vi "calculate bearing example.vi"() -> ()   [LabVIEW 2011]
uses:
  <vilib>/robotics/Controls/Compass Indicator/Compass Indicator.xctl
  <vilib>/express/express arith-compare/Formula/XNode/ExpressFormulaBlockNode.xnode
panel:
  out "Result 2":dbl
  out "Result":dbl
  in  "stop":bool
  in  "Dlong2":dbl format="%#_16g"
  in  "Dlat2":dbl format="%#_16g"
  in  "Dlong1":dbl format="%#_16g"
  in  "Dlat1":dbl format="%#_16g"
  out "Final Bearing":dbl(xcontrol)
  out "Initial Bearing":dbl(xcontrol)
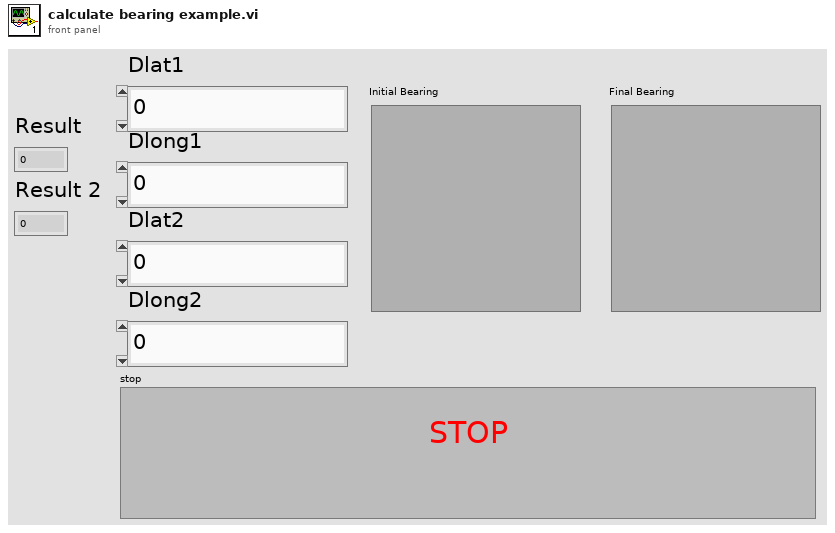
[diagram p1: front panel]
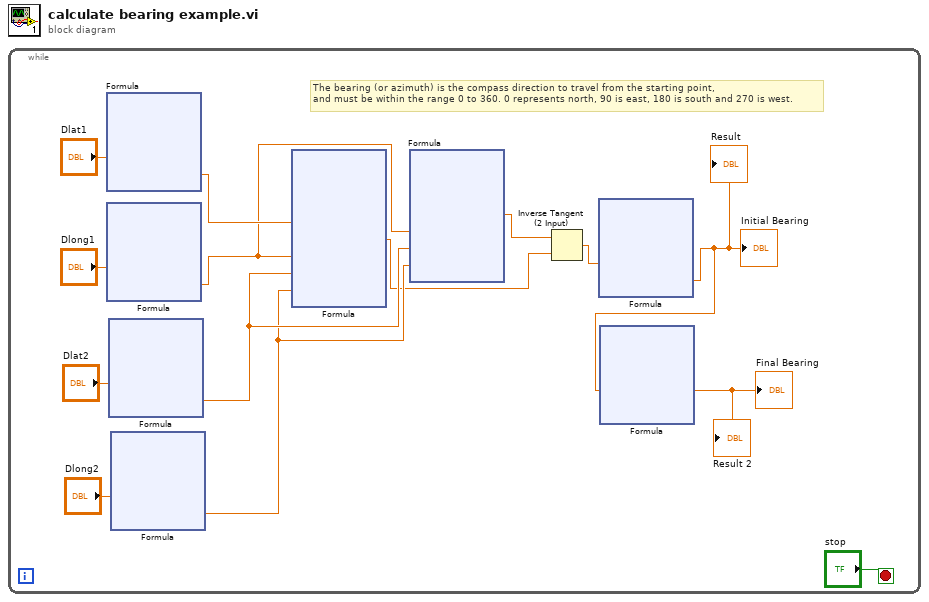
[diagram p0: block diagram]
diagram:
  n1 = while {
    stop <- "stop" stop-if-true
    # "The bearing (or azimuth) is the compass direction to travel from the starting point,\nand must be within the range 0 to 360. 0 represents north, 90 is east, 180 is south and 270 is west."
    n2 = xnode "Formula"("Dlat1"="Dlat1") -> ("Result"=w14:dbl)  [unwired: 1 in, 1 out]
    n3 = xnode "Formula"("Dlong1"="Dlong1") -> ("Result"=w13:dbl)  [unwired: 1 in, 1 out]
    n4 = xnode "Formula"("Dlat2"="Dlat2") -> ("Result"=w12:dbl)  [unwired: 1 in, 1 out]
    n5 = xnode "Formula"("Dlong2"="Dlong2") -> ("Result"=w11:dbl)  [unwired: 1 in, 1 out]
    n6 = xnode "Formula"("lat1"=w14, "long1"=w13, "lat2"=w12, "long2"=w11) -> ("Result"=w9:dbl)  [unwired: 1 in, 1 out]
    n7 = xnode "Formula"("long1"=w13, "lat2"=w12, "long2"=w11) -> ("Result"=w10:dbl)  [unwired: 1 in, 1 out]
    n8 = Inverse Tangent (2 Input)(1:w9, 2:w10) -> (0:w7:dbl)
    n9 = xnode "Formula"("rad"=w7) -> ("Result"=w1:dbl)  [unwired: 1 in, 1 out]
    "Initial Bearing" <- w1
    "Result" <- w1
    n10 = xnode "Formula"("theata"=w1) -> ("Result"=→"Final Bearing" →"Result 2":dbl)  [unwired: 1 in, 1 out]
  }
